vi "Module Top Level VI.vi"(8 "error in":errorcluster) -> (0 "error out":errorcluster)   [LabVIEW 2018, in "Error Handler.lvlib"]
doc: "This is the top level of the error handler module (a free running module of the Car WAsh simulator). \n\nIt is closed using a user event. It communicates with the other modules using a queue based API which has comms modules that can be swapped if required."
uses:
  Error Handler.lvlib
  Private Controls/Module Data Cluster.ctl
  Private Controls/Module Action.ctl
  Public Controls/error cluster.ctl
  User Events/controls/Actions.ctl
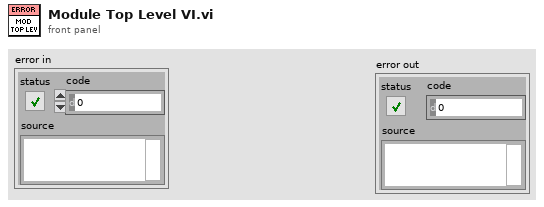
[diagram p1: front panel]
types:
  T1 = typedef "Error Handler.lvlib/error cluster.ctl" = cluster{"error level":enum16{"Minor", "Wash Cycloe", "System Error"}, "description":string}
  T2 = typedef "Actions.ctl" = enum16{"Get", "Create", "Destroy"}
  T3 = typedef "Error Handler.lvlib/Module Data Cluster.ctl" = cluster{"Variant":variant, "action":T4}
  T4 = typedef "Error Handler.lvlib/Module Action.ctl" = enum16{"error", "exit", "init", "Handle Error"}
  T5 = cluster{"Variant":variant, "action":enum16{"error", "exit", "init"}}
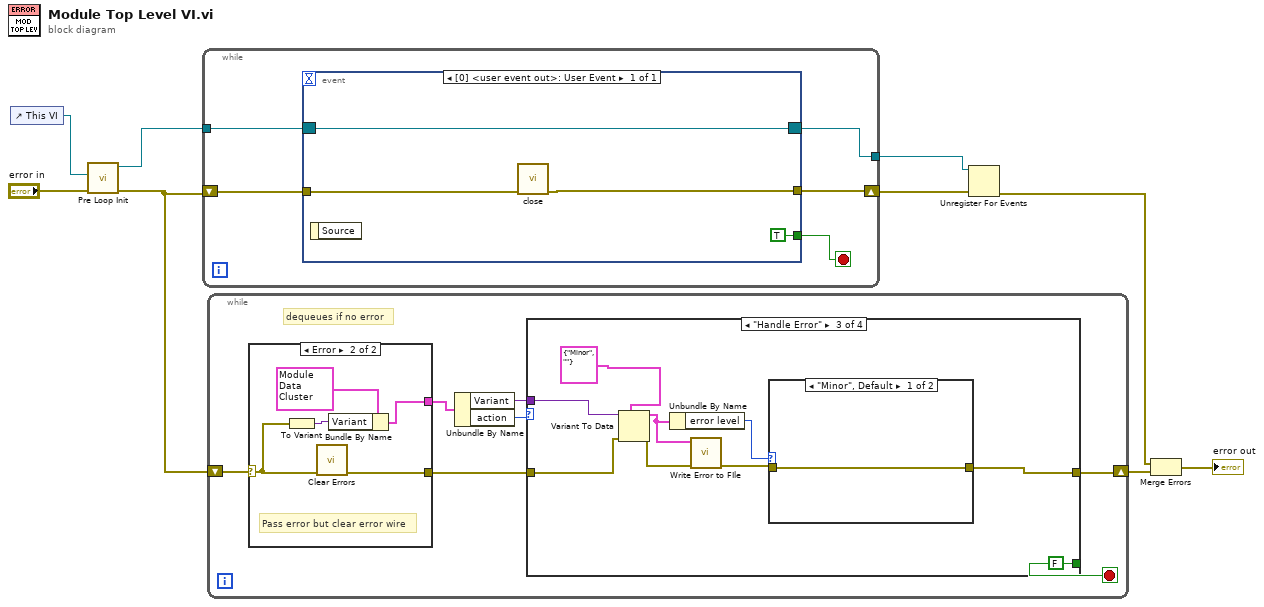
[diagram p0: block diagram]
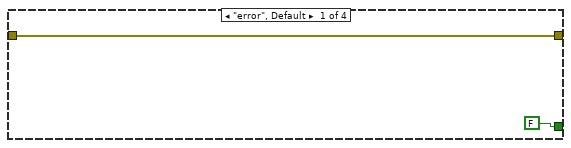
[diagram p2: hidden frame]
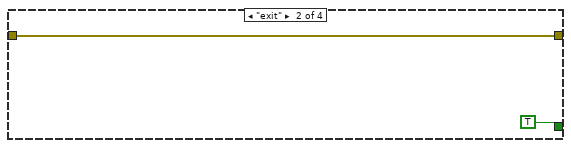
[diagram p3: hidden frame]
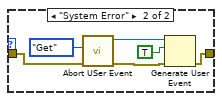
[diagram p4: hidden frame]
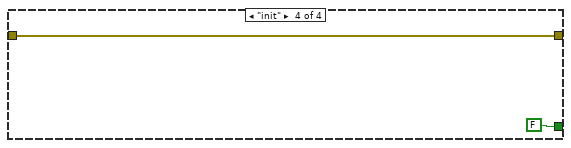
[diagram p5: hidden frame]
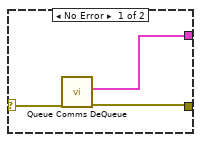
[diagram p6: hidden frame]
diagram:
  n1 = control-ref of="This VI"() -> (w9:refnum<vi>)
  n2 = call "Pre Loop Init.vi"("error in"="error in", "Ref In"=w9) -> ("error out"=w6:errorcluster, "Event Registration Refnum"=w8:refnum<event-registration>)  [unwired: 8 in]
  n3 = while {
    shift-right: [w13] -> w5
    shift-left: w6 -> [w14]
    tunnel: w8 -> [w12]
    tunnel: [w10] -> w4
    stop <- w11 stop-if-true
    n4 = event shown="[0] <user event out>: User Event" {
      selector: w12 -> [w15]
      dyn-events: [w15] -> w10
      timeout: _ -> [_]
      tunnel: w14 -> [w18]
      tunnel: [w17] -> w13
      tunnel: [TRUE] -> w11
      event User Event {
        n5 = event-data() -> ()  [unwired: 1 in, 1 out]
        n6 = call "close.vi"("error in"=w18) -> ("error out"=w17:errorcluster)  [unwired: 10 in]
      }
    }
  }
  n7 = while {
    shift-right: [w21] -> w3
    shift-left: w6 -> [w25]
    stop <- w19 stop-if-true
    # "dequeues if no error"
    n8 = case shown="Error" w25 {
      selector: w25 -> [w50 w55]
      tunnel: [w49 w51] -> w24
      tunnel: [w48 w54] -> w20
      frame No Error {
        n9 = call "Queue Comms DeQueue.vi"("error in"=w50) -> ("error out"=w48:errorcluster, "element"=w49:T5)  [unwired: 9 in]
      }
      frame Error {
        # "Pass error but clear error wire"
        n10 = To Variant(anything=w55) -> (Variant=w52:variant)
        n11 = call <vilib>:"Clear Errors.vi"("error in (no error)"=w55) -> ("error out"=w54:errorcluster)  [unwired: 5 in, 1 out]
        n12 = Bundle By Name(cluster=T3 {"Variant"=variant, "action"=enum."error"} ("element"), "Variant"=w52) -> (w51:T3)
      }
    }
    n13 = Unbundle By Name(w24) -> ("Variant"=w22:variant, "action"=w23:T4)
    n14 = case shown="\"Handle Error\"" w23 {
      tunnel: w22 -> [_ _ w38 _]
      tunnel: [w27 w29 w32 w47] -> w21
      tunnel: w20 -> [w27 w29 w37 w47]
      tunnel: [FALSE TRUE FALSE FALSE] -> w19
      frame "error", Default {
      }
      frame "exit" {
      }
      frame "Handle Error" {
        n15 = Variant To Data(error in=w37, type=T1 {"error level"=enum."Minor", "description"=""} ("error Cluster"), Variant=w38) -> (data=w34:T1, error out=w35:errorcluster)
        n16 = Unbundle By Name(w34) -> ("error level"=w33:enum16{"Minor", "Wash Cycloe", "System Error"})
        n17 = call "Write Error to FIle.vi"("error in"=w35, "error Cluster"=w34) -> ("error out"=w31:errorcluster)  [unwired: 9 in]
        n18 = case shown="\"Minor\", Default" w33 {
          tunnel: w31 -> [w39 w43]
          tunnel: [w39 w41] -> w32
          frame "Minor", Default {
          }
          frame "System Error" {
            n19 = call "Abort USer Event.vi"("error in"=w43, "Enum"=Actions."Get") -> ("error out"=w42:errorcluster, "user event out"=w40:refnum<user-event>)  [unwired: 8 in]
            n20 = Generate User Event(user event=w40, event data cluster=TRUE ("event data"), error in=w42) -> (error out=w41:errorcluster)  [unwired: 1 in, 1 out]
          }
        }
      }
      frame "init" {
      }
    }
  }
  n21 = Unregister For Events(event registration refnum=w4, error in=w5) -> (error out=w1:errorcluster)
  n22 = Merge Errors(w1, w3) -> (→"error out":errorcluster)
